vi "ni579x Wait for Lock.vi"(0 "Register Bus":refnum<class "ni579x Register Bus v1 Host.lvclass">=refnum, 1 "scope":string(combo)="PLL", 9 "timeout [s]":dbl=10.0, 11 "Error In":errorcluster) -> (4 "Register Bus (out)":refnum<class "ni579x Register Bus v1 Host.lvclass">, 15 "Error Out":errorcluster)   [LabVIEW 2013]
doc: "Waits for the specified circuit to complete its configuration and report a successful lock to the supplied reference.\n\n<B>Input Parameters</B>\n\n<B>Register Bus</B> The Register Bus object created by the ni579x Open VI and used as the session handle for the NI-579x Configuration Design Library.\n\n<B>scope</B> The circuit to wait for... \"PLL\" for the reference clock circuit and \"LO1\" for the local oscillator.\n\n<B>timeout [s]</B> How long to wait, in seconds.\n\n<B>Output Parameters</B>\n\n<B>Register Bus (out)</B> The Register Bus object created by the ni579x Open VI and used as the session handle for the NI-579x Configuration Design Library."
uses:
  <instrlib>/ni579x/Register Bus/v1/Host/ni579x Register Bus v1 Host.lvclass
  <instrlib>/ni579x/Config/v1/Shared/Types/ni579x Required FPGA Interface Reference.ctl
  <vilib>/rvi/interface/common/niFpgaWaitOnOcc.vi
  <vilib>/Utility/error.llb/Error Cluster From Error Code.vi
  <vilib>/rvi/errors/niLvFpgaAdjustHostInterfaceError.vi
  <vilib>/rvi/interface/nirviReadWriteControl/nirviReadWriteControl.xnode
  NiFpgaLv.dll
  <vilib>/rvi/interface/Simulation/niFpgaSimulationCallBeginRW.vi
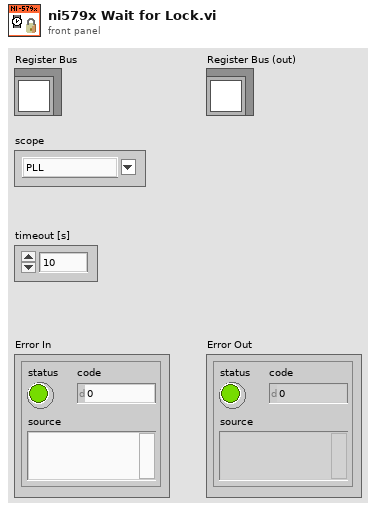
[diagram p1: front panel]
types:
  T1 = typedef "ni579x Required FPGA Interface Reference.ctl" = refnum<k20>
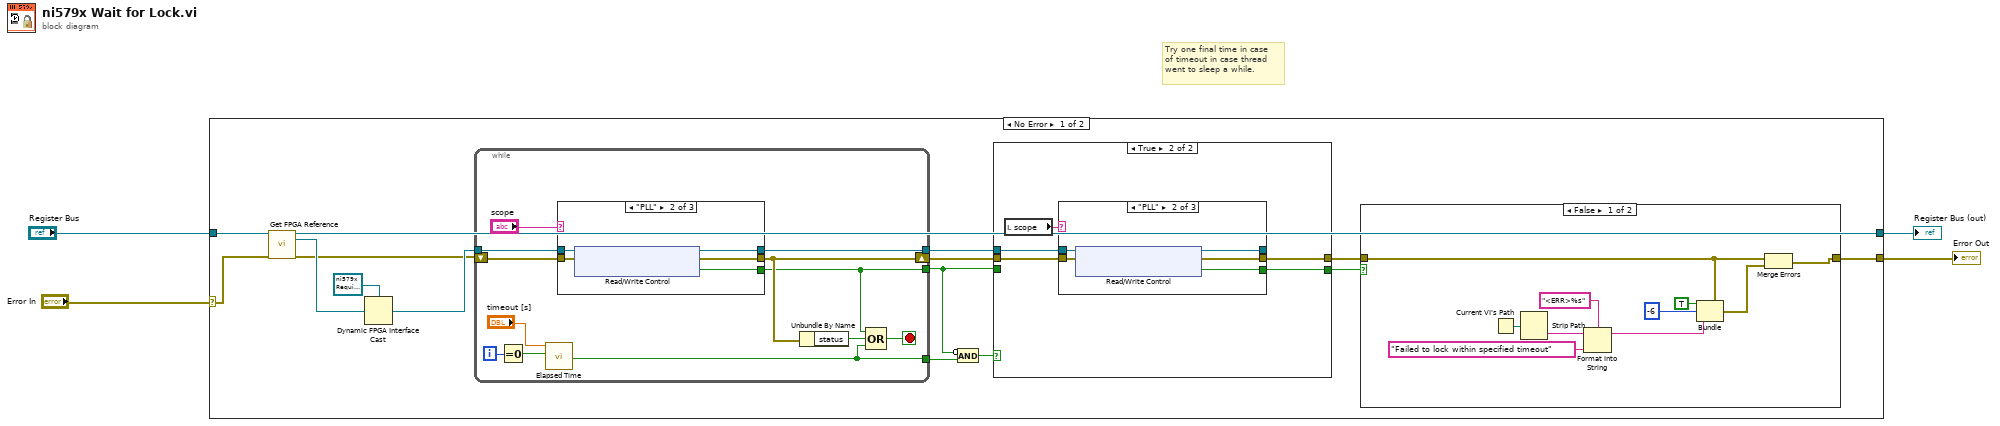
[diagram p0: block diagram]
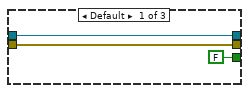
[diagram p3: hidden frame]
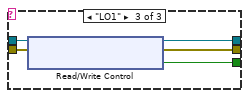
[diagram p4: hidden frame]
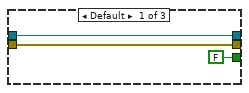
[diagram p6: hidden frame]
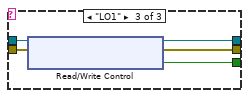
[diagram p7: hidden frame]
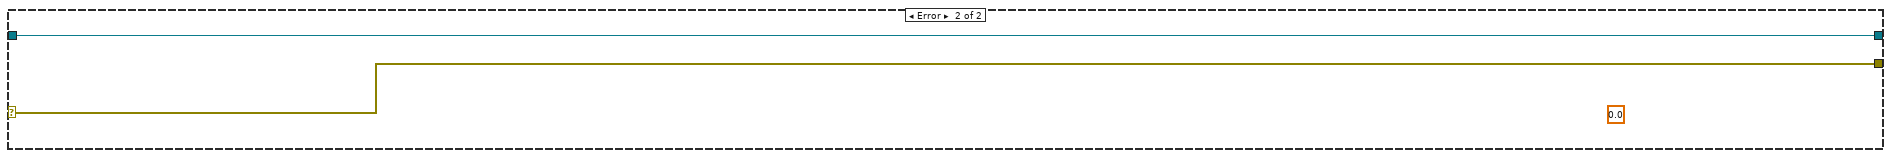
[diagram p8: hidden frame]
diagram:
  # "Try one final time in case\nof timeout in case thread\nwent to sleep a while."
  n1 = case shown="No Error" "Error In" {
    selector: "Error In" -> [w18 w77]
    tunnel: [w9 w77] -> w3
    tunnel: "Register Bus" -> [w19 w76]
    tunnel: [w8 w76] -> w1
    frame No Error {
      n2 = call <instrlib>:"Get FPGA Reference.vi"("session in"=w19, "error in"=w18) -> ("session out"=w8:refnum<class "ni579x Register Bus v1 Host.lvclass">, "fpga ref"=w17:refnum<k20>, "error out"=w15:errorcluster)  [unwired: 11 in]
      n3 = Dynamic FPGA Interface Cast(Session In=T1 refnum ("Type"), Type=w17) -> (Session Out=w16:T1)
      n4 = while {
        tunnel: w16 -> [w56]
        shift-right: [w52] -> w12
        shift-left: w15 -> [w55]
        tunnel: [w59] -> w14
        tunnel: [w54] -> w6
        tunnel: [w51] -> w7
        i -> [w61]
        stop <- w60 stop-if-true
        n5 = Equal To 0?(x=w61) -> (x = 0?=w62:bool)
        n6 = call "Elapsed Time"("Time Target (s)"="timeout [s]", "Reset"=w62) -> ("Time has Elapsed"=w59:bool)  [unwired: 10 in, 7 out]
        n7 = case shown="\"PLL\"" "scope" {
          tunnel: w56 -> [w65 w70 w75]
          tunnel: w55 -> [w64 w69 w74]
          tunnel: [w64 w68 w73] -> w52
          tunnel: [w65 w67 w72] -> w54
          tunnel: [FALSE ("IO Module\\Secondary LO Locked") w66 w71] -> w51
          frame Default {
          }
          frame "PLL" {
            n8 = xnode "Read/Write Control"("FPGA VI Reference In"=w70, "error in"=w69) -> ("FPGA VI Reference Out"=w67:T1, "error out"=w68:errorcluster, "IO Module\\PLL Locked"=w66:bool)
          }
          frame "LO1" {
            n9 = xnode "Read/Write Control"("FPGA VI Reference In"=w75, "error in"=w74) -> ("FPGA VI Reference Out"=w72:T1, "error out"=w73:errorcluster, "IO Module\\LO Locked"=w71:bool)
          }
        }
        n10 = Unbundle By Name(w52) -> ("status"=w53:bool)
        n11 = Compound Arithmetic op=OR(w51, w53, w59) -> (w60:bool)
      }
      n12 = Compound Arithmetic op=AND(invert w7, w14) -> (w13:bool)
      n13 = case shown="True" w13 {
        tunnel: w12 -> [w21 w25]
        tunnel: [w20 w23] -> w11
        tunnel: [w21 w24] -> w10
        tunnel: w7 -> [w20 _]
        tunnel: w6 -> [_ w26]
        frame False {
        }
        frame True {
          n14 = local read "scope"() -> (w22:string)
          n15 = case shown="\"PLL\"" w22 {
            tunnel: w26 -> [w29 w34 w39]
            tunnel: w25 -> [w28 w33 w38]
            tunnel: [w28 w32 w37] -> w24
            tunnel: [w29 w31 w36] -> _
            tunnel: [FALSE ("IO Module\\Secondary LO Locked") w30 w35] -> w23
            frame Default {
            }
            frame "PLL" {
              n16 = xnode "Read/Write Control"("FPGA VI Reference In"=w34, "error in"=w33) -> ("FPGA VI Reference Out"=w31:T1, "error out"=w32:errorcluster, "IO Module\\PLL Locked"=w30:bool)
            }
            frame "LO1" {
              n17 = xnode "Read/Write Control"("FPGA VI Reference In"=w39, "error in"=w38) -> ("FPGA VI Reference Out"=w36:T1, "error out"=w37:errorcluster, "IO Module\\LO Locked"=w35:bool)
            }
          }
        }
      }
      n18 = case shown="False" w11 {
        tunnel: w10 -> [w41 w50]
        tunnel: [w40 w50] -> w9
        frame False {
          n19 = Current VI's Path() -> (path=w48:path)
          n20 = Strip Path(path=w48) -> (name=w47:string)  [unwired: 1 out]
          n21 = Format Into String(format string="<ERR>%s", initial string=w47, "Failed to lock within specified timeout" ("input 1")) -> (resulting string=w46:string)  [unwired: 1 in, 1 out]
          n22 = Bundle(cluster=w41, "status"=TRUE, "code"=-6, "source"=w46) -> (w45:errorcluster)
          n23 = Merge Errors(w41, w45) -> (w40:errorcluster)
        }
        frame True {
        }
      }
    }
    frame Error {
      (unwired) 0.0 ("coerced attenuation [dB]")
    }
  }
  "Register Bus (out)" <- w1
  "Error Out" <- w3
